vi "SetIntValue.vi"(3 "error in (no error)":errorcluster, 4 "nValue":i64, 5 "strName":string, 6 "nInputHandle":u64) -> (0 "error out":errorcluster, 1 "GX_STATUS":i32, 2 "nOutputHandle":u64)   [LabVIEW 2016, in "GxLVLib.lvlib"]
uses:
  GxLVLib.lvlib
  GxIAPI.dll
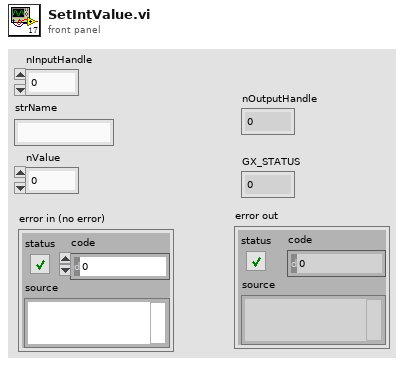
[diagram p1: front panel]
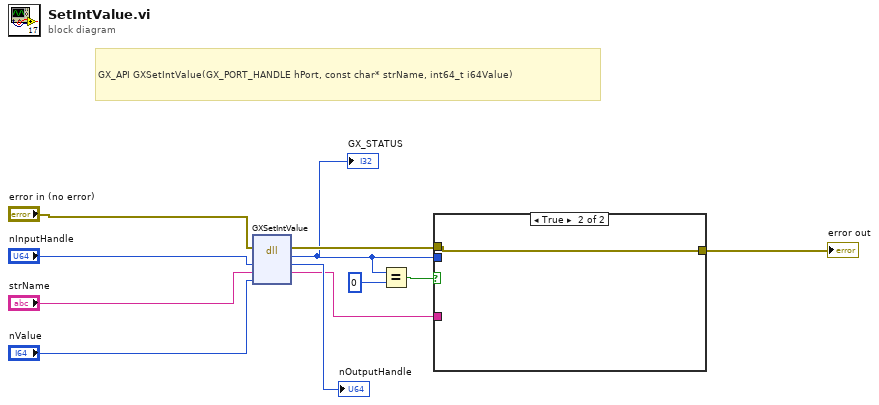
[diagram p0: block diagram]
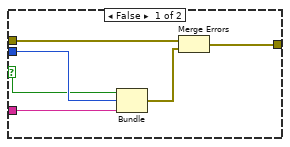
[diagram p2: hidden frame]
diagram:
  # "GX_API GXSetIntValue(GX_PORT_HANDLE hPort, const char* strName, int64_t i64Value)"
  n1 = dll-call lib="GxIAPI.dll" fn="GXSetIntValue"(error in="error in (no error)", "phDevice"="nInputHandle", "strName"="strName", "i64Value"="nValue") -> (error out=w9:errorcluster, "GX_STATUS"=w5:i32, "phDevice"=→"nOutputHandle":i64, "strName"=w6:string)  [unwired: 3 in, 1 out]
  "GX_STATUS" <- w5
  n2 = Equal?(x=w5, y=0) -> (x = y?=w7:bool)
  n3 = case shown="True" w7 {
    selector: w7 -> [w14 _]
    tunnel: w9 -> [w17 w18]
    tunnel: w5 -> [w15 _]
    tunnel: w6 -> [w13 _]
    tunnel: [w12 w18] -> w4
    frame False {
      n4 = Bundle(w14, "GX_STATUS"=w15, "strName"=w13) -> (w16:cluster{bool, "GX_STATUS":i32, "strName":string})  [unwired: 1 in]
      n5 = Merge Errors(w17, w16) -> (w12:errorcluster)
    }
    frame True {
    }
  }
  "error out" <- w4
